vi "GUI_BELLA_Plasma1_LP_Controller.vi"() -> ()   [LabVIEW 2011]
uses:
  GUI_Template/GUI_master/tcp_new_data_event.ctl
  GUI_Template/GUI_master/tcp new data cluster.ctl
panel:
  in  "stop":bool
  in  "PressureSetPoint::1":dbl=0.001 caption="Pressure Set Point" min=0.0 max=0.0 format="%_4f"
  in  "PressureReading::1":dbl=0.001 caption="Pressure Reading" min=0.0 max=0.0 format="%_4p"
  in  "GUIdevice 1":string="BELLA_Plasma1_LP_Controller"
  out "tcp data event":T1
  out "error IO 2":errorcluster
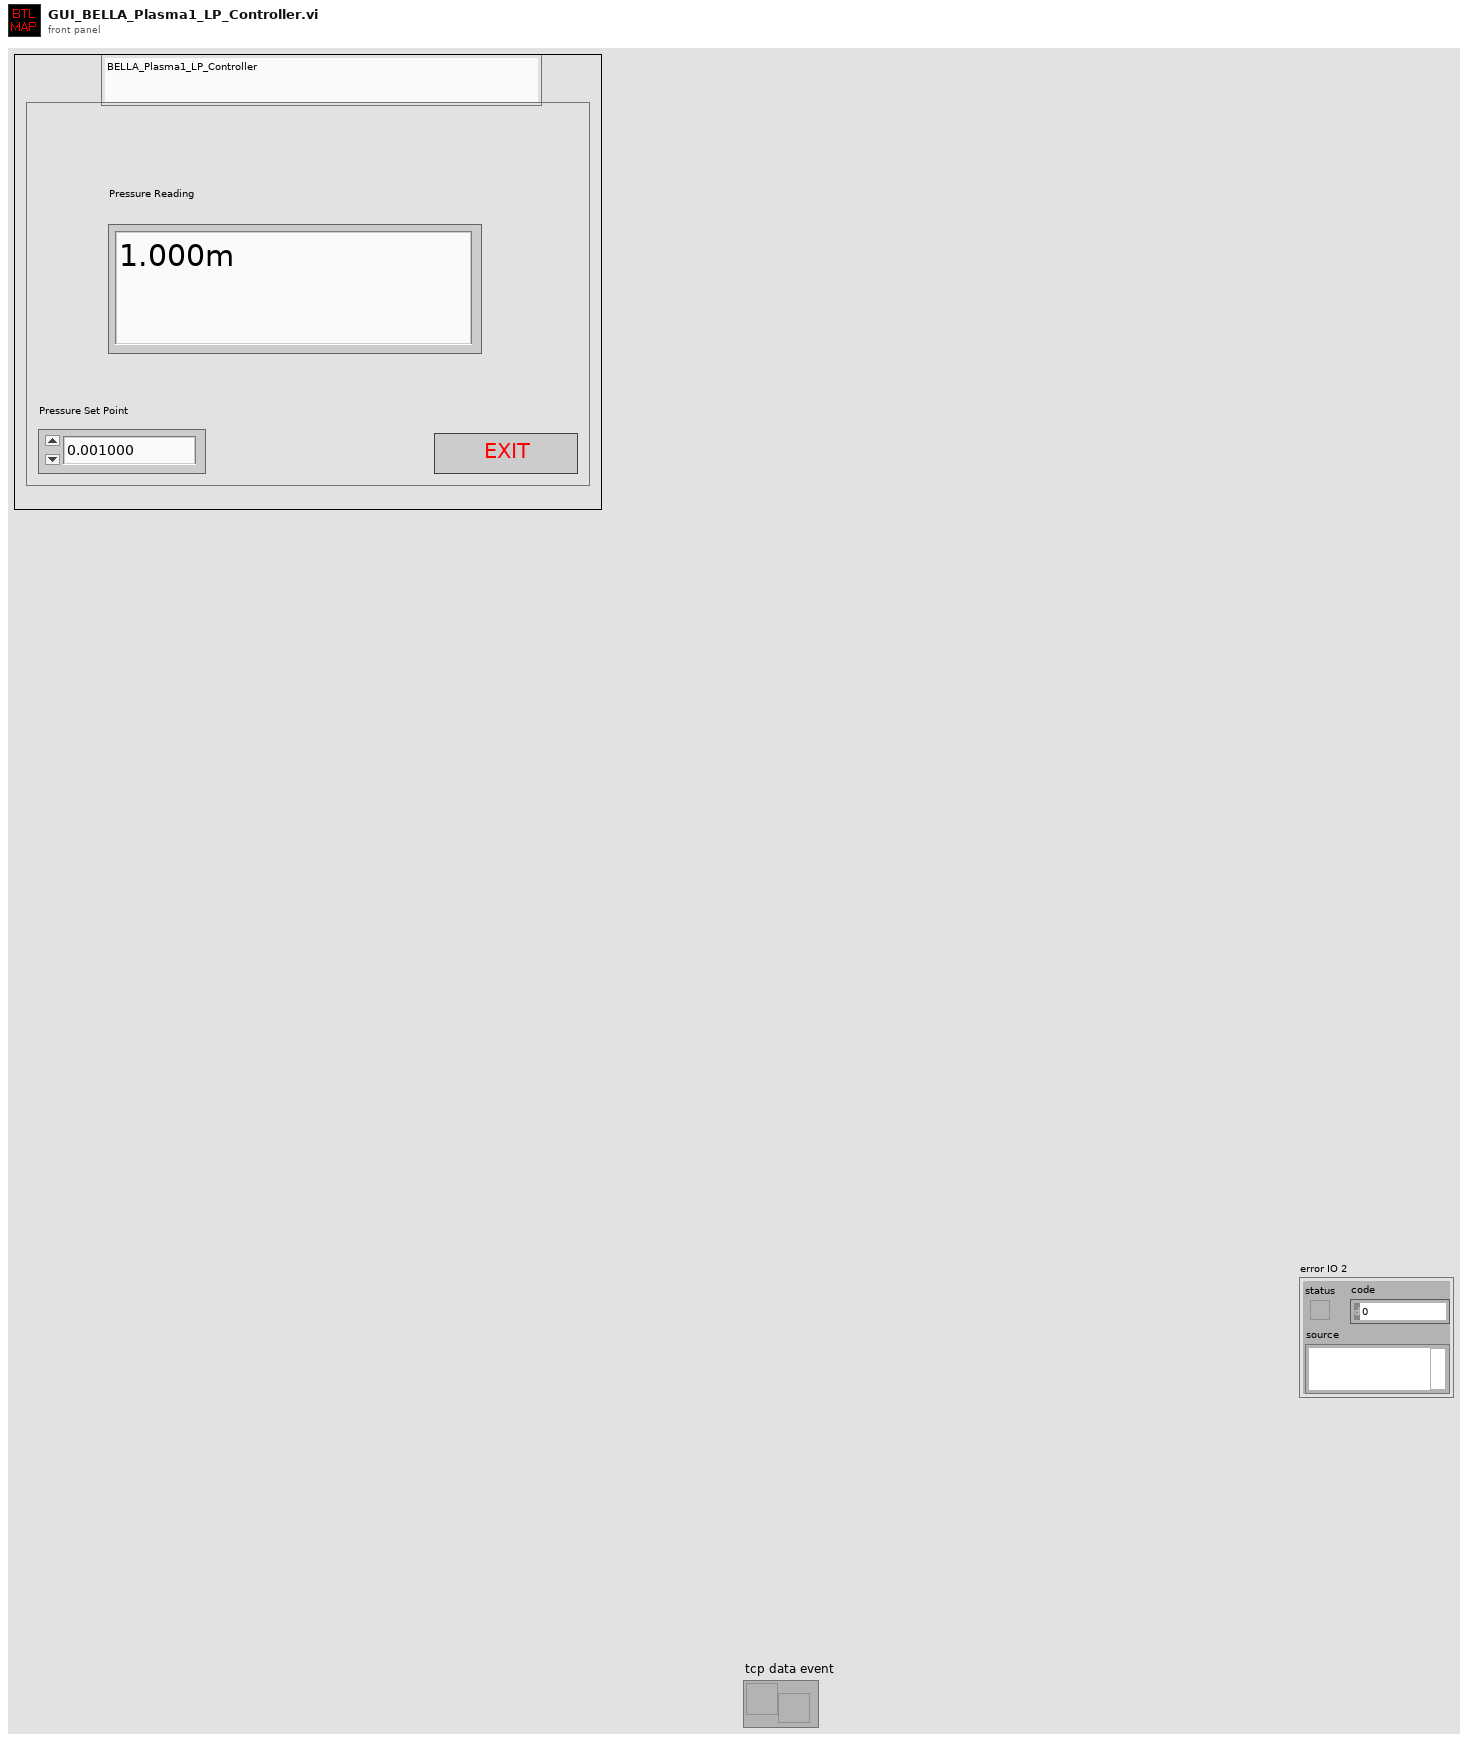
[diagram p1: front panel]
types:
  T1 = typedef "tcp_new_data_event.ctl" = refnum<user-event>
  T2 = typedef "tcp new data cluster.ctl" = cluster{"EventEnum":enum16{"new data", "connection status update"}, "Device name":string}
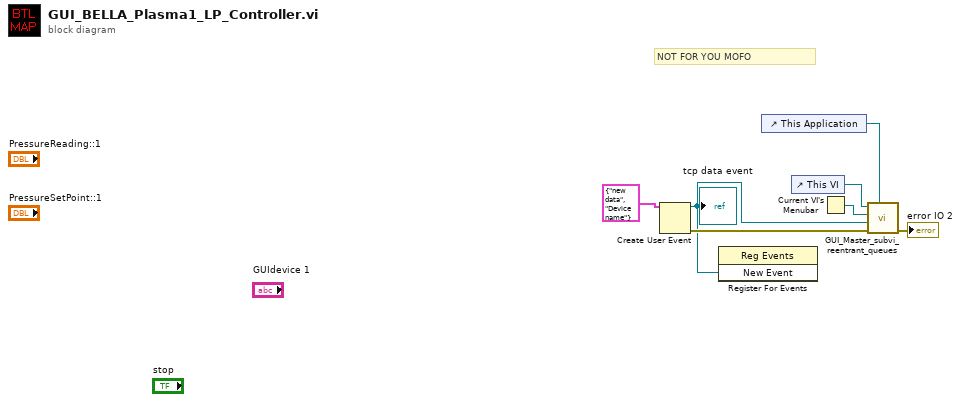
[diagram p0: block diagram]
diagram:
  # "NOT FOR YOU MOFO"
  n1 = Create User Event(user event datatype=T2 {"EventEnum"=enum."new data", "Device name"="Device name"} ("New Event")) -> (user event=w2:refnum<user-event>, error out=w3:errorcluster)  [unwired: 1 in]
  "tcp data event" <- w2
  n2 = register-events(w2) -> ()  [unwired: 2 in, 2 out]
  n3 = control-ref of="This Application"() -> (w1:refnum<vi>)
  n4 = control-ref of="This VI"() -> (w6:refnum<vi>)
  n5 = Current VI's Menubar() -> (w5:refnum<k9>)
  n6 = call "GUI_Master_subvi_reentrant_queues.vi"("This Application"=w1, "error in (no error)"=w3, "tcp data event"=w2, "Caller menu reference"=w5, "Caller VI ref"=w6) -> ("error out"=→"error IO 2":errorcluster)  [unwired: 6 in]
